vi "drivetrain_get_encoders.vi"() -> (1 "Avg Velocity (Ft/Sec)":dbl, 2 "Velocity (in/sec)":cluster{"Left":dbl, "Right":dbl}, 3 "Distance (in)":cluster{"Left":dbl, "Right":dbl})   [LabVIEW 2011]
panel:
  out "error out 2":errorcluster
  out "error out":errorcluster
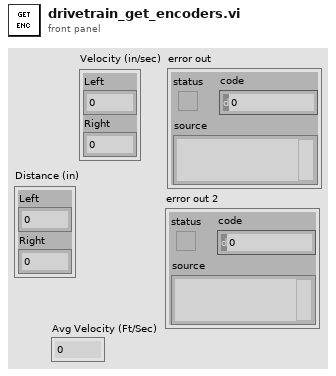
[diagram p1: front panel]
types:
  T1 = typedef "WPI_EncoderDevRef.ctl" = cluster{"DevStatus":errorcluster, "EncoderIndex":T2, "CounterIndex":T3, "DistancePerCount":dbl, "Decoding Type":T4}
  T2 = typedef "FPGA_EncoderIdx.ctl" = enum8{"Enc 0", "Enc 1", "Enc 2", "Enc 3", "Invalid"}
  T3 = typedef "FPGA_CounterCtrSystemIndex.ctl" = enum8{"Ctr 0", "Ctr 1", "Ctr 2", "Ctr 3", "Ctr 4", "Ctr 5", "Ctr 6", "Ctr 7", "Invalid"}
  T4 = typedef "WPI_EncoderType.ctl" = enum16{"1x", "2x", "4x"}
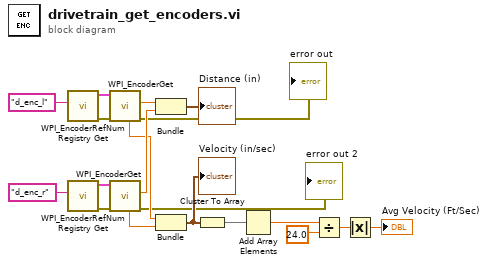
[diagram p0: block diagram]
diagram:
  n1 = call <vilib>:"WPI_EncoderRefNum Registry Get.vi"("refnum name"="d_enc_l") -> ("error out"=w4:errorcluster, "EncoderDevRef"=w17:T1)  [unwired: 9 in]
  n2 = call <vilib>:"WPI_EncoderRefNum Registry Get.vi"("refnum name"="d_enc_r") -> ("error out"=w3:errorcluster, "EncoderDevRef"=w16:T1)  [unwired: 9 in]
  n3 = call <vilib>:"WPI_EncoderGet.vi"("error in (no error)"=w4, "EncoderDevRef"=w17) -> ("error out"=→"error out":errorcluster, "Distance"=w14:dbl, "Rate"=w12:dbl)  [unwired: 4 in, 3 out]
  n4 = call <vilib>:"WPI_EncoderGet.vi"("error in (no error)"=w3, "EncoderDevRef"=w16) -> ("error out"=→"error out 2":errorcluster, "Distance"=w13:dbl, "Rate"=w11:dbl)  [unwired: 4 in, 3 out]
  n5 = Bundle("Distance"=w14, "Distance"=w13) -> (→"Distance (in)":cluster{"Distance":dbl, "Distance":dbl})  [unwired: 1 in]
  n6 = Bundle("Rate"=w12, "Rate"=w11) -> (w10:cluster{"Rate":dbl, "Rate":dbl})  [unwired: 1 in]
  "Velocity (in/sec)" <- w10
  n7 = Cluster To Array(cluster=w10) -> (array=w9:dbl[])
  n8 = Add Array Elements(numeric array=w9) -> (sum=w8:dbl)
  n9 = Divide(x=w8, y=24.0) -> (x/y=w6:dbl)
  n10 = Absolute Value(x=w6) -> (abs(x)=→"Avg Velocity (Ft/Sec)":dbl)
